vi "Push button.vi"() -> (1 "Push Button":T1)   [LabVIEW 2020]
uses:
  Galobal variable_TI.vi
panel:
  in  "Cluster":T1
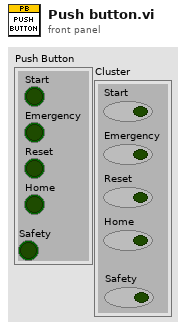
[diagram p1: front panel]
types:
  T1 = cluster{"Start":bool, "Emergency ":bool, "Reset":bool, "Home":bool, "Safety":bool}
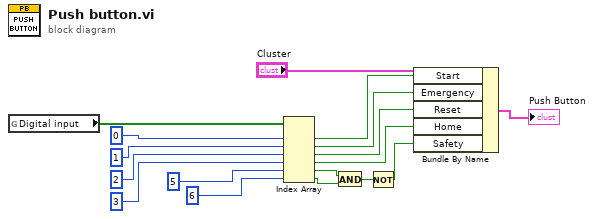
[diagram p0: block diagram]
diagram:
  n1 = global read "Galobal variable_TI.vi" "Digital input"() -> (w13:bool[])
  n2 = Index Array(array=w13, index #1=0 ("index"), index #2=1 ("index"), index #3=2 ("index"), index #4=3 ("index"), index #5=5 ("index"), index #6=6 ("index")) -> (element #1=w11:bool, element #2=w10:bool, element #3=w9:bool, element #4=w8:bool, element #5=w4:bool, element #6=w3:bool)
  n3 = And(x=w4, y=w3) -> (x .and. y?=w2:bool)
  n4 = Not(x=w2) -> (.not. x?=w1:bool)
  n5 = Bundle By Name(cluster="Cluster", "Start"=w11, "Emergency"=w10, "Reset"=w9, "Home"=w8, "Safety"=w1) -> (→"Push Button":T1)
